vi "Do.vi"(8 "error in (no error)":errorcluster, 10 "Actor in":refnum<class "Actor.lvclass">, 11 "SetAOTask Msg in":refnum<class "SetAOTask Msg.lvclass">) -> (0 "error out":errorcluster, 2 "Actor out":refnum<class "Actor.lvclass">)   [LabVIEW 2015, in "IO Device.lvlib" / "SetAOTask Msg.lvclass"]
doc: "(<B>Filename</B>: Actor Framework.lvlib:Message.lvclass:Do.vi)\n\nDefines what a message does when it is received by an actor. Generally, a message instructs an actor to invoke one of its methods. By default, this method does nothing. A child class must override it to define behavior. Create a child class by using the Actor Framework Message Maker dialog box."
uses:
  SetAOTask Msg.lvclass
  IO Device/IO Device.lvclass
  <vilib>/ActorFramework/Actor/Actor.lvclass
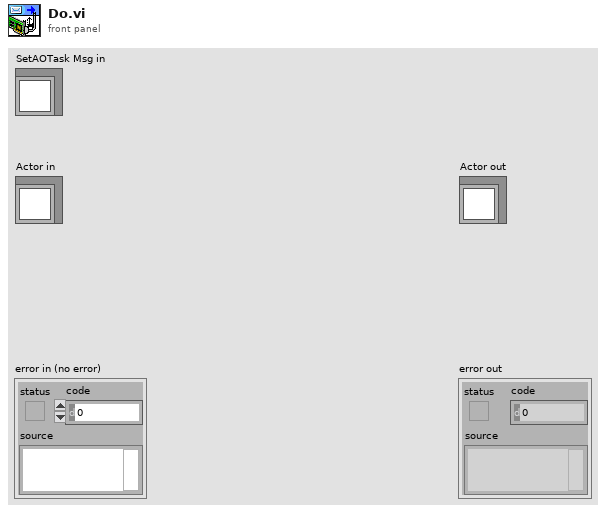
[diagram p1: front panel]
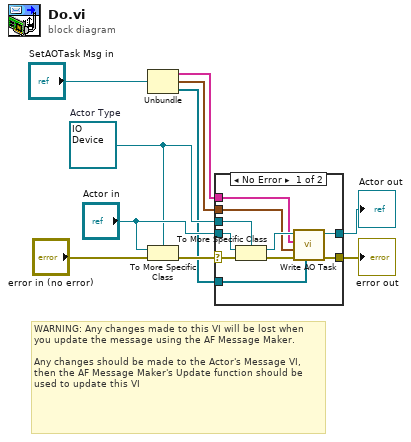
[diagram p0: block diagram]
diagram:
  w5 = refnum<class "IO Device.lvclass"> refnum  # Actor Type
  # "WARNING: Any changes made to this VI will be lost when you update the message using the AF Message Maker.\n\nAny changes should be made to the Actor's Message VI, then the AF Message Maker's Update function should be used to update this VI"
  n1 = Unbundle("SetAOTask Msg in") -> (w4:tag[], w3:waveform(dbl)[], w2:refnum<class "AOChConfig.lvclass">[])
  n2 = To More Specific Class(target class=w5, reference="Actor in", error in="error in (no error)") -> (error out=w9:errorcluster)  [unwired: 1 out]
  n3 = case shown="No Error" w9 {
    selector: w9 -> [w20 w22]
    tunnel: [w15 w22] -> w8
    tunnel: [w14 w21] -> w7
    tunnel: "Actor in" -> [w19 w21]
    tunnel: w5 -> [w18 _]
    tunnel: w4 -> [w13 _]
    tunnel: w3 -> [w12 _]
    tunnel: w2 -> [w11 _]
    frame No Error {
      n4 = To More Specific Class ("Actor Cast")(target class=w18, reference=w19, error in=w20) -> (specific class reference=w17:refnum<class "IO Device.lvclass">, error out=w16:errorcluster)
      n5 = call-dynamic "Write AO Task.vi"("AOChConfigs"=w11, "error in (no error)"=w16, "AO Waveforms"=w12, "AO DAQChannels"=w13, "IO Device in"=w17) -> ("error out"=w15:errorcluster, "IO Device out"=w14:refnum<class "IO Device.lvclass">)  [unwired: 5 in]
    }
    frame Error {
    }
  }
  "error out" <- w8
  "Actor out" <- w7
